vi "gfitsio-get-num-hdus.vi"(8 "error in (no error)":errorcluster, 11 "gfits refnum":T1) -> (0 "error out":errorcluster, 2 "number of hdus":i32, 3 "dup gfits refnum":T1)   [LabVIEW 2019, in "gfitsio.lvlib"]
doc: "Return the total number of HDUs in the FITS file. This returns the number of completely defined HDUs in the file. If a new HDU has just been added to the FITS file, then that HDU will only be counted if it has been closed, or if data has been written to the HDU. The current HDU remains unchanged by this VI."
uses:
  gfitsio.lvlib
  gfitsio-refnum.ctl
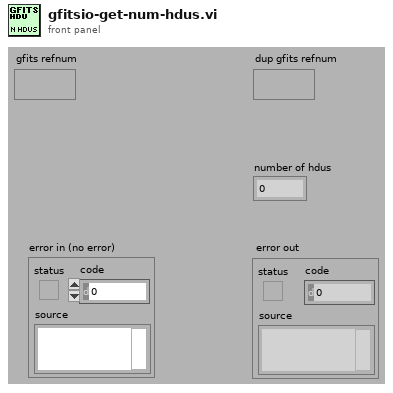
[diagram p1: front panel]
types:
  T1 = typedef "gfitsio.lvlib/gfitsio-refnum.ctl" = refnum<k1>
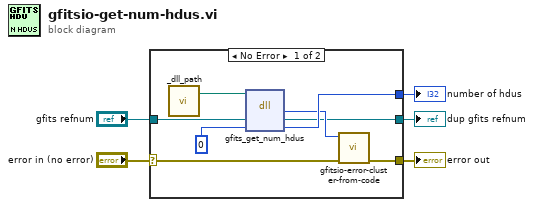
[diagram p0: block diagram]
diagram:
  n1 = case shown="No Error" "error in (no error)" {
    selector: "error in (no error)" -> [w11 w15]
    tunnel: [w10 w15] -> w5
    tunnel: "gfits refnum" -> [w8 w14]
    tunnel: [w9 w14] -> w3
    tunnel: [w13 _] -> w1
    frame No Error {
      n2 = call "_dll_path.vi"() -> ("Path"=w6:path)  [unwired: 1 in]
      n3 = dll-call lib="?" fn="gfits_get_num_hdus"(path in=w6, "refnum"=w8, "numhdus"=0) -> ("return type"=w12:i32, "refnum"=w9:T1, "numhdus"=w13:i32)  [unwired: 2 in, 2 out]
      n4 = call "gfitsio-error-cluster-from-code.vi"("error in (no error)"=w11, "error code"=w12) -> ("error out"=w10:errorcluster)  [unwired: 9 out]
    }
    frame Error {
    }
  }
  "error out" <- w5
  "dup gfits refnum" <- w3
  "number of hdus" <- w1
